vi "Open Client Connection.vi"(8 "error in (no error)":errorcluster, 9 "Port":u16, 10 "address":string, 11 "RemoteControl.STM in":refnum<class "RemoteControl.STM.lvclass">) -> (0 "error out":errorcluster, 3 "RemoteControl.STM out":refnum<class "RemoteControl.STM.lvclass">)   [LabVIEW 2019, in "RemoteControl.STM.lvclass"]
uses:
  RemoteControl.STM.lvclass
  <vilib>/NI/STM/TCP/TCP Read Options.ctl
  RemoteControl.STM.lvclass/RemoteControl.STM.ctl
  <vilib>/NI/STM/TCP/Read Meta Data (TCP Clst).vi
  <vilib>/NI/STM/TCP/Read Meta Data (TCP Ref).vi
  RemoteControl/RemoteControl.lvclass
  <vilib>/NI/STM/NI STM.lvlib
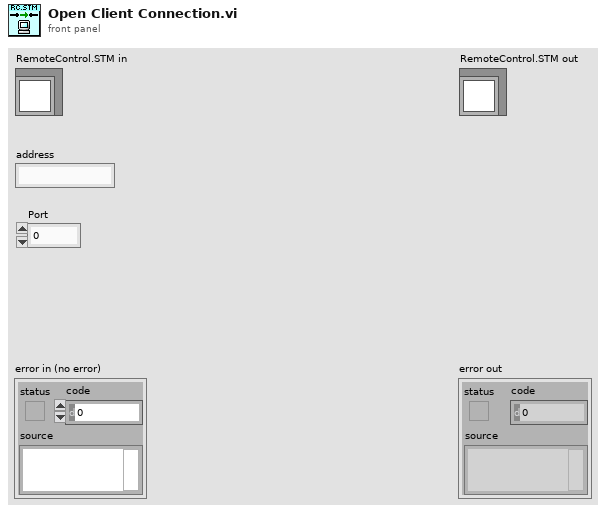
[diagram p1: front panel]
types:
  T1 = typedef "NI STM.lvlib/TCP Read Options.ctl" = cluster{"ignore timeout error":bool, "timeout ms (1000)":i32}
  T2 = typedef "NI STM.lvlib/TCP Connection Info.ctl" = cluster{"connection ID":refnum<k5>, "meta data":T3[]}
  T3 = typedef "NI STM.lvlib/MetaDataElement.ctl" = string
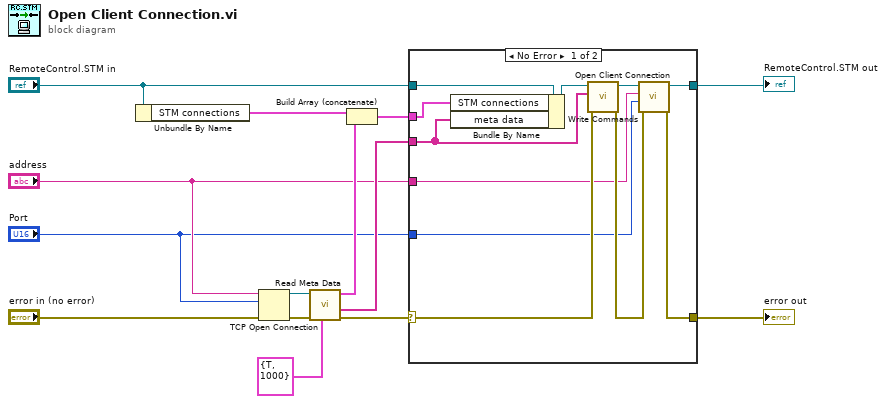
[diagram p0: block diagram]
diagram:
  n1 = Unbundle By Name("RemoteControl.STM in") -> ("STM connections"=w5:T2[])
  n2 = TCP Open Connection(address="address", remote port or service name="Port", error in (no error)="error in (no error)") -> (connection ID=w13:refnum<k5>, error out=w14:errorcluster)  [unwired: 2 in]
  n3 = call-poly <vilib>:"Read Meta Data.vi"("options"=T1 {"ignore timeout error"=TRUE, "timeout ms (1000)"=1000}, "error in"=w14, "connection ID"=w13) -> ("error out"=w4:errorcluster, "meta data"=w8:T3[], "connection info out"=w12:T2)  [unwired: 6 in]
  n4 = Build Array (concatenate)(w5, w12) -> (w9:T2[])
  n5 = case shown="No Error" w4 {
    selector: w4 -> [w23 w27]
    tunnel: [w19 w27] -> w10
    tunnel: w9 -> [w15 _]
    tunnel: w8 -> [w18 _]
    tunnel: "RemoteControl.STM in" -> [w24 w26]
    tunnel: [w21 w26] -> w3
    tunnel: "address" -> [w17 _]
    tunnel: "Port" -> [w16 _]
    frame No Error {
      n6 = Bundle By Name(cluster=w24, "STM connections"=w15, "meta data"=w18) -> (w25:refnum<class "RemoteControl.STM.lvclass">)
      n7 = call-dynamic "Write Commands.vi"("error in (no error)"=w23, "Commands"=w18, "RemoteControl in"=w25) -> ("error out"=w20:errorcluster, "RemoteControl out"=w22:refnum<class "RemoteControl.STM.lvclass">)  [unwired: 7 in]
      n8 = call-parent "Open Client Connection.vi"("error in (no error)"=w20, "Port"=w16, "address"=w17, "RemoteControl in"=w22) -> ("error out"=w19:errorcluster, "RemoteControl out"=w21:refnum<class "RemoteControl.STM.lvclass">)  [unwired: 6 in]
    }
    frame Error {
    }
  }
  "error out" <- w10
  "RemoteControl.STM out" <- w3
